vi "JSON structure validation.vi"(8 "error in (no error)":errorcluster, 9 "JSON path":string, 10 "Compare\nvariant":variant, 11 "Reference\nvariant":variant) -> (0 "error out":errorcluster, 2 "Continue?":bool, 3 "Element name":string)   [LabVIEW 2015]
uses:
  <vilib>/Utility/Data Type/NI_Data Type.lvlib
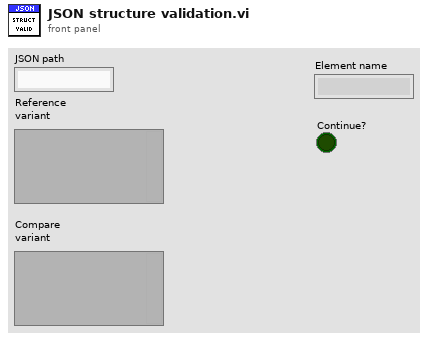
[diagram p1: front panel]
types:
  T1 = typedef "NI_Data Type.lvlib/Data Type.ctl" = enum8{"Invalid Type", "Void", "I8", "I16", "I32", "I64", "U8", "U16", "U32", "U64", "Single Float", "Double Float", "Extended Float", "Single Complex", "Double Complex", "Extended Complex", "Enum U8", "Enum U16", "Enum U32", "Enum U64", "Single Float With Unit", "Double Float With Unit", "Extended Float With Unit", "Single Complex with Unit", "Double Complex with Unit", "Extended Complex with Unit", "Boolean", "String", "Path", "Picture", "Tag", "Array", "Cluster", "Variant", "LV Variant", "Waveform", "Timestamp", "Digital Waveform", "Digital Data", "ExpressData", "Refnum", "External Data", "VI", "Poly VI", "LabVIEW Class Instance", "Fixed Point"}
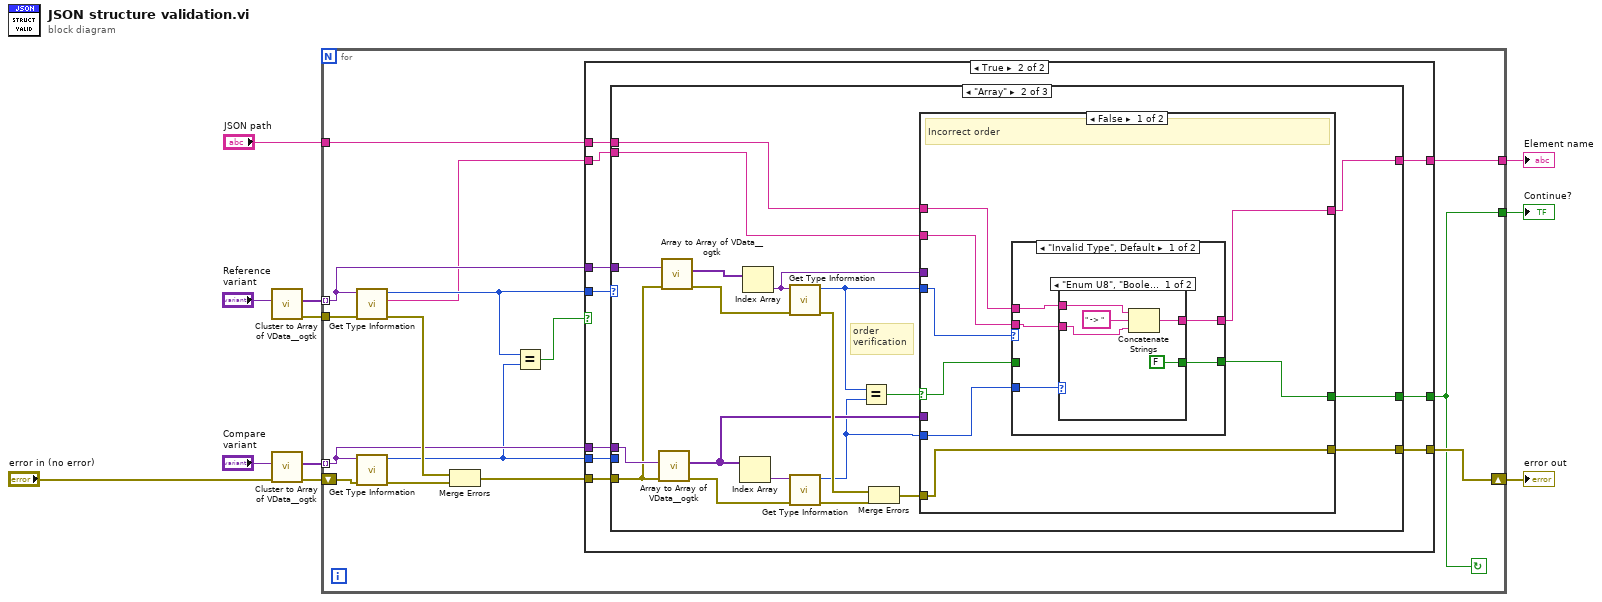
[diagram p0: block diagram]
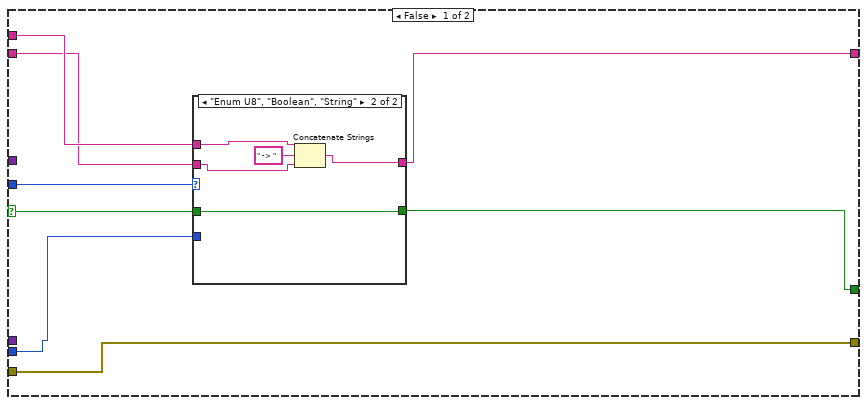
[diagram p2: hidden frame]
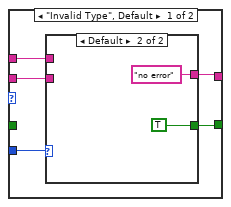
[diagram p3: hidden frame]
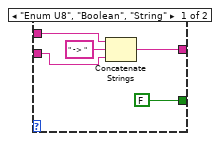
[diagram p4: hidden frame]
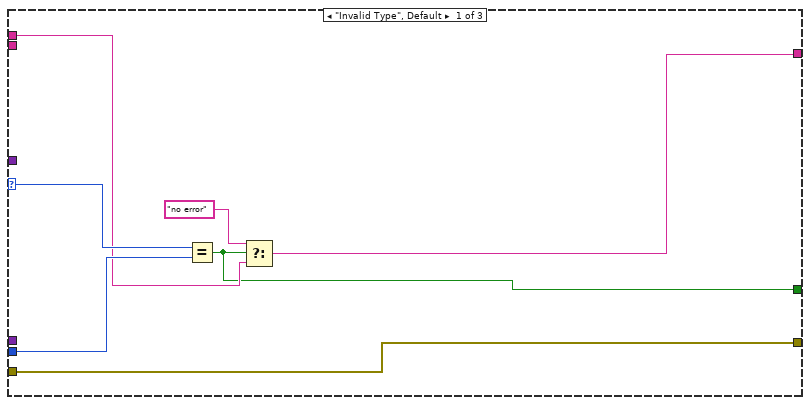
[diagram p5: hidden frame]
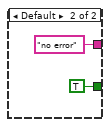
[diagram p6: hidden frame]
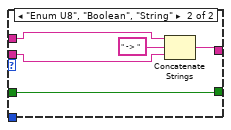
[diagram p7: hidden frame]
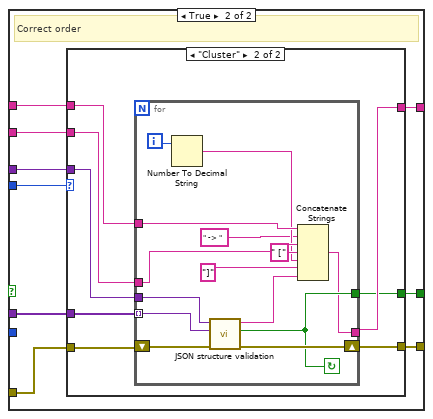
[diagram p8: hidden frame]
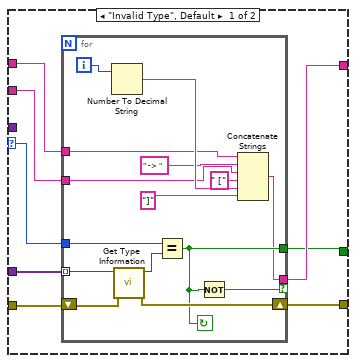
[diagram p9: hidden frame]
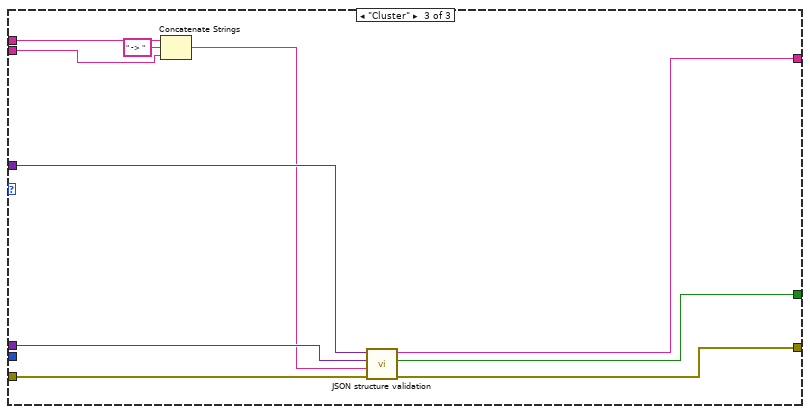
[diagram p10: hidden frame]
diagram:
  n1 = call <userlib>:"Cluster to Array of VData__ogtk.vi"("Cluster"="Reference\nvariant") -> ("error out"=w9:errorcluster, "Array of VData"=w8:variant[])  [unwired: 9 in]
  n2 = call <userlib>:"Cluster to Array of VData__ogtk.vi"("error in (no error)"="error in (no error)", "Cluster"="Compare\nvariant") -> ("error out"=w11:errorcluster, "Array of VData"=w10:variant[])  [unwired: 8 in]
  n3 = for {
    tunnel: w10 -> [w19] mode=indexing
    tunnel: w9 -> [w25]
    tunnel: w8 -> [w20] mode=indexing
    tunnel: [w17] -> w7
    shift-right: [w16] -> w3
    shift-left: w11 -> [w26]
    tunnel: [w13] -> w2
    tunnel: "JSON path" -> [w12]
    stop <- w13 continue-if-true
    n4 = call <vilib>:"Get Type Information.vi"("error in (no error)"=w25, "Variant"=w20) -> ("error out"=w23:errorcluster, "Name"=w18:string, "Type"=w24:T1)  [unwired: 5 in, 2 out]
    n5 = call <vilib>:"Get Type Information.vi"("error in (no error)"=w26, "Variant"=w19) -> ("error out"=w22:errorcluster, "Type"=w15:T1)  [unwired: 5 in, 3 out]
    n6 = Merge Errors(w23, w22) -> (w21:errorcluster)
    n7 = Equal?(x=w24, y=w15) -> (x = y?=w14:bool)
    n8 = case shown="True" w14 {
      selector: w14 -> [w32 _]
      tunnel: w24 -> [w33 w61]
      tunnel: w21 -> [w34 w60]
      tunnel: w20 -> [_ w59]
      tunnel: w19 -> [_ w58]
      tunnel: w18 -> [w28 w52]
      tunnel: [w27 w57] -> w17
      tunnel: [w34 w56] -> w16
      tunnel: w15 -> [w30 w55]
      tunnel: [w31 w54] -> w13
      tunnel: w12 -> [w29 w53]
      frame False {
        n9 = case shown="\"Enum U8\", \"Boolean\", \"String\"" w33 {
          tunnel: w32 -> [_ w51]
          tunnel: [w39 w51] -> w31
          tunnel: w30 -> [w38 _]
          tunnel: w29 -> [w37 w49]
          tunnel: w28 -> [w36 w48]
          tunnel: [w35 w47] -> w27
          frame "Invalid Type", Default {
            n10 = case shown="Default" w38 {
              tunnel: [FALSE TRUE] -> w39
              tunnel: w37 -> [w42 _]
              tunnel: w36 -> [w41 _]
              tunnel: [w40 "no error"] -> w35
              frame "Enum U8", "Boolean", "String" {
                n11 = Concatenate Strings(w42, " -> " ("string"), w41) -> (w40:string)
              }
              frame Default {
              }
            }
          }
          frame "Enum U8", "Boolean", "String" {
            n12 = Concatenate Strings(w49, " -> " ("string"), w48) -> (w47:string)
          }
        }
      }
      frame True {
        n13 = case shown="\"Array\"" w61 {
          selector: w61 -> [w68 _ _]
          tunnel: w60 -> [w63 w86 w177]
          tunnel: w59 -> [_ w88 w176]
          tunnel: w58 -> [_ w87 w175]
          tunnel: w53 -> [w65 w74 w171]
          tunnel: [w64 w73 w173] -> w57
          tunnel: [w63 w72 w174] -> w56
          tunnel: w55 -> [w67 _ _]
          tunnel: [w62 w71 w172] -> w54
          tunnel: w52 -> [_ w70 w169]
          frame "Invalid Type", Default {
            n14 = Equal?(x=w68, y=w67) -> (x = y?=w62:bool)
            n15 = Select(t="no error", s=w62, f=w65) -> (s? t:f=w64:string)
          }
          frame "Array" {
            # "order\nverification"
            n16 = call <userlib>:"Array to Array of VData__ogtk.vi"("error in (no error)"=w86, "MultiD Array"=w87) -> ("error out"=w83:errorcluster, "1D Array of Variants"=w75:variant[])  [unwired: 8 in]
            n17 = call <userlib>:"Array to Array of VData__ogtk.vi"("error in (no error)"=w86, "MultiD Array"=w88) -> ("error out"=w84:errorcluster, "1D Array of Variants"=w85:variant[])  [unwired: 8 in]
            n18 = Index Array(array=w75) -> (element=w78:variant)  [unwired: 1 in]
            n19 = Index Array(array=w85) -> (element=w76:variant)  [unwired: 1 in]
            n20 = call <vilib>:"Get Type Information.vi"("error in (no error)"=w84, "Variant"=w76) -> ("error out"=w80:errorcluster, "Type"=w77:T1)  [unwired: 5 in, 3 out]
            n21 = call <vilib>:"Get Type Information.vi"("error in (no error)"=w83, "Variant"=w78) -> ("error out"=w81:errorcluster, "Type"=w69:T1)  [unwired: 5 in, 3 out]
            n22 = Equal?(x=w77, y=w69) -> (x = y?=w82:bool)
            n23 = Merge Errors(w80, w81) -> (w79:errorcluster)
            n24 = case shown="False" w82 {
              selector: w82 -> [w92 _]
              tunnel: w79 -> [w96 w121]
              tunnel: w77 -> [w94 w122]
              tunnel: w76 -> [_ w120]
              tunnel: w75 -> [_ w119]
              tunnel: w74 -> [w91 w118]
              tunnel: [w89 w117] -> w73
              tunnel: [w96 w116] -> w72
              tunnel: [w95 w115] -> w71
              tunnel: w70 -> [w90 w114]
              tunnel: w69 -> [w93 _]
              frame False {
                # "Incorrect order"
                n25 = case shown="\"Invalid Type\", Default" w94 {
                  tunnel: w92 -> [_ w113]
                  tunnel: [w101 w113] -> w95
                  tunnel: w93 -> [w100 _]
                  tunnel: w91 -> [w99 w111]
                  tunnel: w90 -> [w98 w110]
                  tunnel: [w97 w109] -> w89
                  frame "Invalid Type", Default {
                    n26 = case shown="\"Enum U8\", \"Boolean\", \"String\"" w100 {
                      tunnel: [FALSE TRUE] -> w101
                      tunnel: w99 -> [w105 _]
                      tunnel: w98 -> [w104 _]
                      tunnel: [w102 "no error"] -> w97
                      frame "Enum U8", "Boolean", "String" {
                        n27 = Concatenate Strings(w105, " -> " ("string"), w104) -> (w102:string)
                      }
                      frame Default {
                      }
                    }
                  }
                  frame "Enum U8", "Boolean", "String" {
                    n28 = Concatenate Strings(w111, " -> " ("string"), w110) -> (w109:string)
                  }
                }
              }
              frame True {
                # "Correct order"
                n29 = case shown="\"Cluster\"" w122 {
                  selector: w122 -> [w128 _]
                  tunnel: w121 -> [w129 w153]
                  tunnel: w120 -> [_ w152]
                  tunnel: w119 -> [w130 w151]
                  tunnel: w118 -> [w124 w147]
                  tunnel: [w126 w150] -> w117
                  tunnel: [w127 w149] -> w116
                  tunnel: [w125 w148] -> w115
                  tunnel: w114 -> [w123 w146]
                  frame "Invalid Type", Default {
                    n30 = for {
                      tunnel: w130 -> [w145] mode=indexing
                      shift-right: [w143] -> w127
                      shift-left: w129 -> [w144]
                      tunnel: w128 -> [w141]
                      tunnel: [w131] -> w126 if=w140
                      tunnel: [w139] -> w125
                      tunnel: w124 -> [w133]
                      tunnel: w123 -> [w132]
                      i -> [w134]
                      stop <- w139 continue-if-true
                      n31 = Number To Decimal String(number=w134) -> (decimal integer string=w136:string)  [unwired: 1 in]
                      n32 = call <vilib>:"Get Type Information.vi"("error in (no error)"=w144, "Variant"=w145) -> ("error out"=w143:errorcluster, "Type"=w142:T1)  [unwired: 5 in, 3 out]
                      n33 = Equal?(x=w141, y=w142) -> (x = y?=w139:bool)
                      n34 = Not(x=w139) -> (.not. x?=w140:bool)
                      n35 = Concatenate Strings(w133, " -> " ("string"), w132, " [" ("string"), w136, "]" ("string")) -> (w131:string)
                    }
                  }
                  frame "Cluster" {
                    n36 = for {
                      tunnel: w152 -> [w166]
                      tunnel: w151 -> [w165] mode=indexing
                      tunnel: [w154] -> w150
                      shift-right: [w164] -> w149
                      shift-left: w153 -> [w167]
                      tunnel: [w163] -> w148
                      tunnel: w147 -> [w162]
                      tunnel: w146 -> [w161]
                      i -> [w160]
                      stop <- w163 continue-if-true
                      n37 = Number To Decimal String(number=w160) -> (decimal integer string=w157:string)  [unwired: 1 in]
                      n38 = call "JSON structure validation.vi"("error in (no error)"=w167, "Compare\nvariant"=w165, "Reference\nvariant"=w166) -> ("error out"=w164:errorcluster, "Continue?"=w163:bool, "Element name"=w155:string)  [unwired: 6 in]
                      n39 = Concatenate Strings(w162, " -> " ("string"), w161, " [" ("string"), w157, "]" ("string"), w155) -> (w154:string)
                    }
                  }
                }
              }
            }
          }
          frame "Cluster" {
            n40 = Concatenate Strings(w171, " -> " ("string"), w169) -> (w168:string)
            n41 = call "JSON structure validation.vi"("error in (no error)"=w177, "JSON path"=w168, "Compare\nvariant"=w175, "Reference\nvariant"=w176) -> ("error out"=w174:errorcluster, "Continue?"=w172:bool, "Element name"=w173:string)  [unwired: 5 in]
          }
        }
      }
    }
  }
  "Element name" <- w7
  "error out" <- w3
  "Continue?" <- w2
